vi "Ramp.vi"(7 "Sample Rate":dbl, 9 "Ramp Amplitude":dbl=10.0, 10 "Ramp Duration":dbl=8.0, 11 "Array in":dbl[](array[numeric])) -> (2 "Array out":dbl[](array[numeric]))   [LabVIEW 2016]
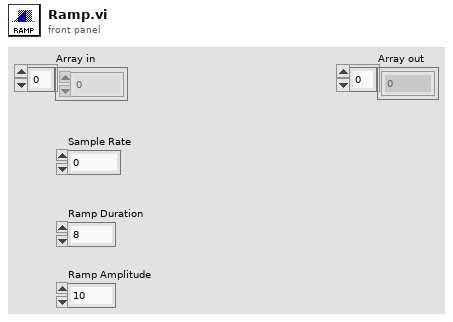
[diagram p1: front panel]
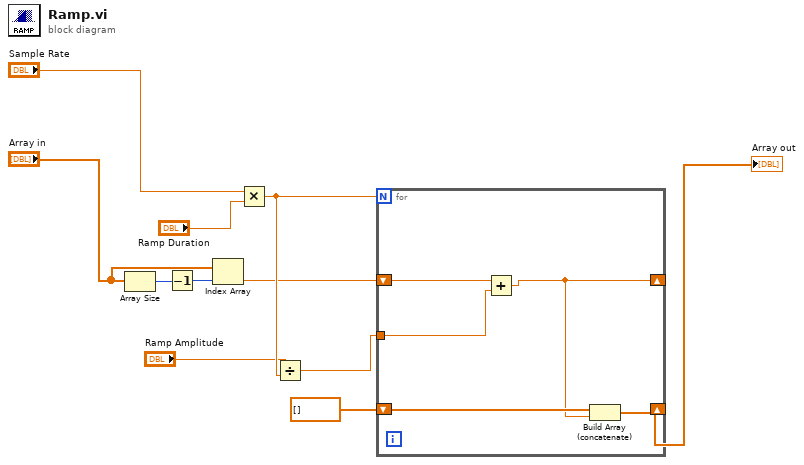
[diagram p0: block diagram]
diagram:
  n1 = Array Size(array="Array in") -> (size(s)=w10:i32)
  n2 = Decrement(x=w10) -> (x-1=w11:i32)
  n3 = Index Array(array="Array in", index=w11) -> (element=w4:dbl)
  n4 = Multiply(x="Sample Rate", y="Ramp Duration") -> (x*y=w8:dbl)
  n5 = Divide(x="Ramp Amplitude", y=w8) -> (x/y=w9:dbl)
  n6 = for {
    N: w8 -> [_]
    shift-right: [w14] -> _
    shift-left: w4 -> [w16]
    shift-right: [w13] -> w2
    shift-left: dbl[] [] -> [w15]
    tunnel: w9 -> [w12]
    n7 = Add(x=w16, y=w12) -> (x+y=w14:dbl)
    n8 = Build Array (concatenate)(w15, w14) -> (w13:dbl[])
  }
  "Array out" <- w2
